vi "DAQ AI.vi"(8 "error in":errorcluster, 10 "Config":T1={"min value"=-5.0, "max value"=5.0, "rate"=1000.0, "samples per channel"=100} {"rate" format="%#_13g"; "max value" format="%#_13g"; "min value" format="%#_13g"}, 11 "Alias":string) -> (0 "error out":errorcluster, 3 "Data":dbl format="%0.2f")   [LabVIEW 2021]
uses:
  Controls/DAQ_Data.ctl
  Controls/Measure Type.ctl
  <vilib>/DAQmx/read.llb/DAQmx Read (Analog 1D DBL 1Chan NSamp).vi
  <vilib>/Analysis/baseanly.llb/Mean (DBL).vi
  <vilib>/DAQmx/create/channels.llb/DAQmx Create Channel (AI-Voltage-Basic).vi
  <vilib>/DAQmx/configure/timing.llb/DAQmx Timing (Sample Clock).vi
  <vilib>/DAQmx/miscellaneous.llb/DAQmx Fill In Error Info.vi
  <vilib>/Analysis/NI_AALBase.lvlib
panel:
  out "Waveform":dbl[](graph)=[-0.14969328897976622, 0.32349620044557026, 0.5157628101443525, 1.0013122959074678, 1.2315744499038668, 1.4925077059236427, 1.74031800286874, 2.183751945554979, 2.4330881679738763, 2.672658467360454, 2.7527695547349467, 3.198950163274026, 3.382976775414289, 3.5392315439313946, 3.6779381694998015, 3.7778862880336925, 3.9722891933957944, 4.208960234382153, 4.282357249671926, 4.408856471449934, 4.758903775139622, 4.6809289834284495, 4.649494918668172, 4.662923062837611, 4.692678609576708, 4.813226722006897, 4.849543748283334, 4.832911160618916, 4.7943052461317786, 4.729453413495285, 4.5121616260261845, 4.557939390240181, 4.373455000457778, 4.2052980132450335, 3.9619129001739557, 3.955656605731376, 3.8218329416791286, 3.6260567033906064, 3.325754570146794, 3.031861323892941, 2.9631946775719475, 2.666707358012635, 2.4730674153874324, 2.192602313303018, 1.7970824304940947, 1.391338847010712, 1.1946470534379101, 0.8291879024628437, 0.716422009949034, 0.2172917874691, 0.0837733085116123, -0.20142216254158146, -0.4588457899716178, -0.7588427381206702, -1.172673726615192, -1.5309610278633992, -1.8555253761406294, -2.1259193700979644, -2.2344126712851344, -2.7416302987762076, -2.8878139591662344, -3.2135990478225045, -3.2667012543107394, -3.6684774315622426, -3.884243293557543, -3.7978759117404706, -4.162266914883877, -4.317911313211463, -4.362010559404279, -4.45188756981109, -4.511246070741905, -4.629505294961394, -4.768364513077182, -4.900051881466109, -4.766991180150762, -4.8594622638630325, -4.852748191778313, -4.67696157719657, -4.690542313913388, -4.814905240028077, -4.582811975463119, -4.543595690786462, -4.317911313211463, -4.217200231940672, -4.073305459761345, -3.9651173436689353, -3.8415173802911466, -3.6178167058320874, -3.3423871578112125, -3.000579851680044, -2.845545823541978, -2.4518570513016145, -2.260963774529252, -2.1114230780968657, -1.8846705526902066, -1.4516129032258065, -1.2085329752494889, -1.0397656178472243, -0.5479598376415296, -0.3032013916440321]
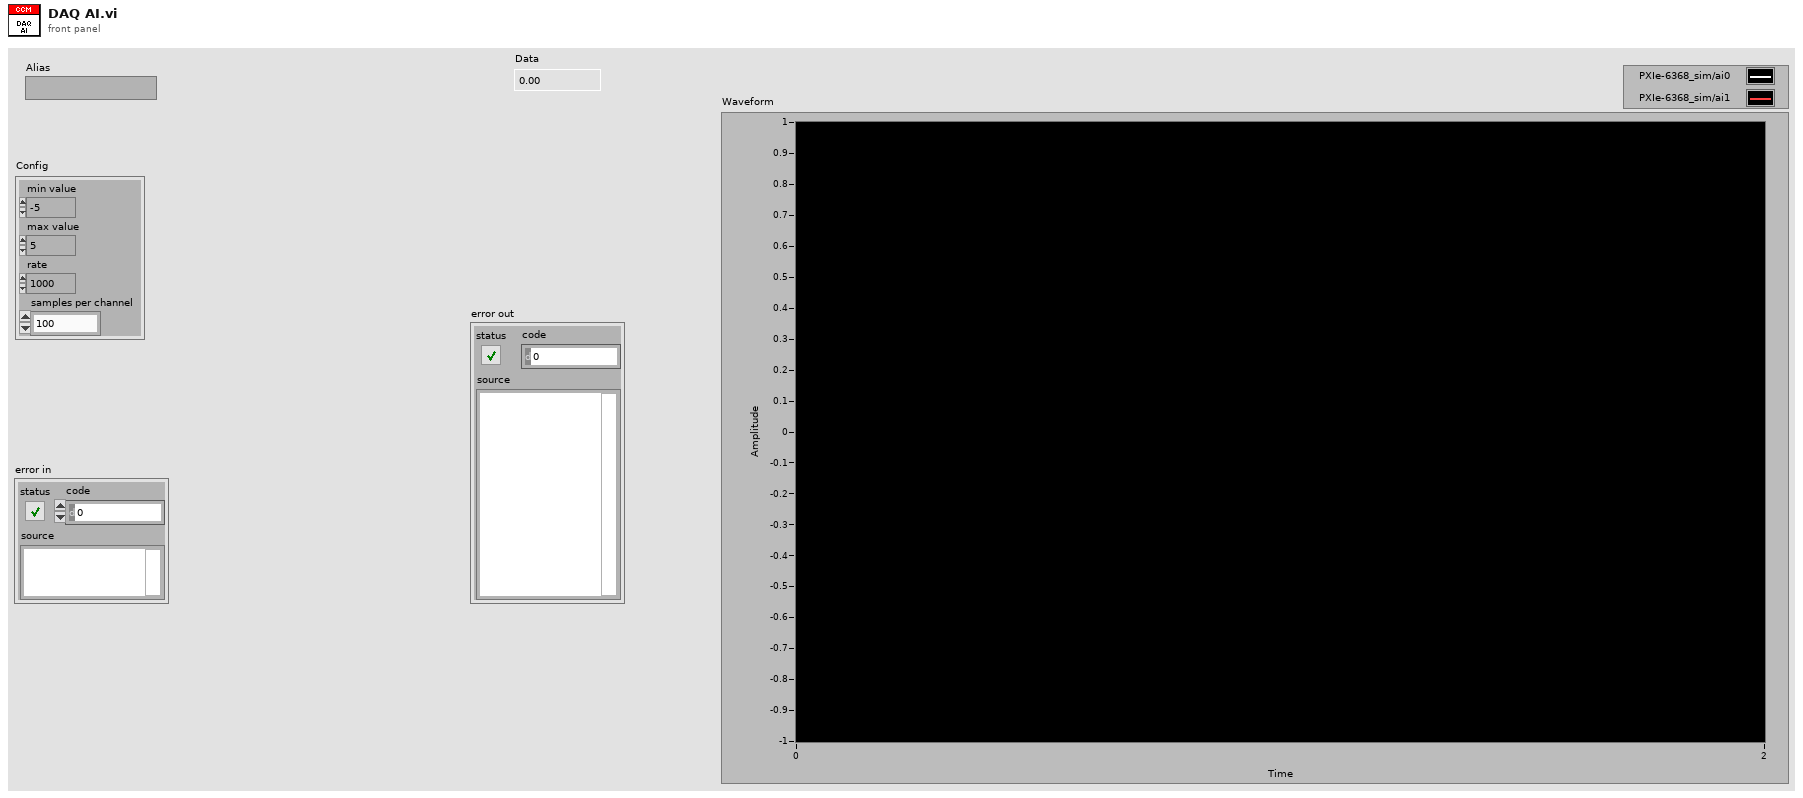
[diagram p1: front panel]
types:
  T1 = cluster{"min value":dbl, "max value":dbl, "rate":dbl, "samples per channel":i32}
  T2 = typedef "Measure Type.ctl" = enum16{"Analog_In", "Analog_Out", "Digital_In", "Digital_Out", "Switch", "NI_DMM"}
  T3 = typedef "DAQ_Data.ctl" = cluster{"Alias":string, "DAQ Ch":string}
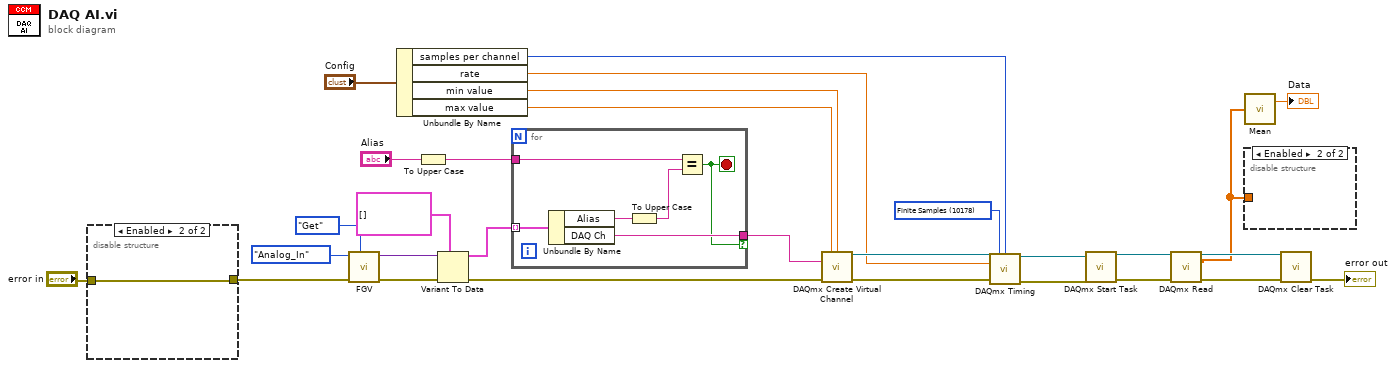
[diagram p0: block diagram]
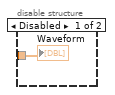
[diagram p2: hidden frame]
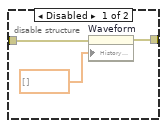
[diagram p3: hidden frame]
diagram:
  w20 = 10178 items=["Finite Samples"=10178, "Continuous Samples"=10123, "Hardware Timed Single Point"=12522] ("sample mode")
  n1 = disable-structure shown="Enabled" {
    disable-tunnel: "error in" -> [w31 w33]
    disable-tunnel: [w30 w33] -> w3
    frame Disabled {
      n2 = property on="Waveform" class="WFChart (strict)"(error in=w31, "History Data"=dbl[] []) -> (error out=w30:errorcluster)  [unwired: 1 in, 1 out]
    }
    frame Enabled {
    }
  }
  n3 = call "FGV.vi"("Method (Get)"=enum16{"Get", "Set"}."Get", "error in"=w3, "Name"=Measure_Type."Analog_In") -> ("error out"=w10:errorcluster, "Data out"=w11:variant)  [unwired: 7 in]
  n4 = Unbundle By Name("Config") -> ("samples per channel"=w15:i32, "rate"=w17:dbl, "min value"=w19:dbl, "max value"=w18:dbl)
  n5 = To Upper Case(1:"Alias") -> (0:w1:string)
  n6 = Variant To Data(error in=w10, type=T3[] [], Variant=w11) -> (data=w7:T3[], error out=w8:errorcluster)
  n7 = for {
    tunnel: w7 -> [w39] mode=indexing
    tunnel: [w38] -> w5 if=w35
    tunnel: w1 -> [w37]
    stop <- w35 stop-if-true
    n8 = Unbundle By Name(w39) -> ("Alias"=w36:string, "DAQ Ch"=w38:string)
    n9 = To Upper Case(1:w36) -> (0:w34:string)
    n10 = Equal?(x=w37, y=w34) -> (x = y?=w35:bool)
  }
  n11 = call-poly <vilib>:"DAQmx Create Virtual Channel.vi"("maximum value"=w18, "minimum value"=w19, "physical channels"=w5, "error in"=w8) -> ("task out"=w22:refnum<k21>, "error out"=w24:errorcluster)  [unwired: 10 in]
  n12 = call-poly <vilib>:"DAQmx Timing.vi"("task/channels in"=w22, "sample mode"=w20, "samples per channel"=w15, "rate"=w17, "error in"=w24) -> ("task out"=w21:refnum<k21>, "error out"=w23:errorcluster)  [unwired: 9 in]
  n13 = call <vilib>:"DAQmx Start Task.vi"("task/channels in"=w21, "error in"=w23) -> ("task out"=w27:refnum<k21>, "error out"=w26:errorcluster)  [unwired: 12 in]
  n14 = call-poly <vilib>:"DAQmx Read.vi"("task/channels in"=w27, "error in"=w26) -> ("task out"=w16:refnum<k21>, "data"=w14:dbl[], "error out"=w25:errorcluster)  [unwired: 11 in]
  n15 = call-poly <vilib>:"Mean.vi"("X"=w14) -> ("mean"=→"Data":dbl)  [unwired: 1 out]
  n16 = disable-structure shown="Enabled" {
    disable-tunnel: w14 -> [w40 _]
    frame Disabled {
      "Waveform" <- w40
    }
    frame Enabled {
    }
  }
  n17 = call <vilib>:"DAQmx Clear Task.vi"("task in"=w16, "error in"=w25) -> ("error out"=→"error out":errorcluster)  [unwired: 13 in]
